vi "Page_Source_Add.vi"(4 "ctlReferences":T2, 6 "sourceInclusion":T1, 7 "items to add in":string[](array[string]), 8 "error in (no error)":errorcluster, 9 "send to main dest?":bool, 10 "Project Refnum":refnum<vi>, 11 "AB_Source_Library in":refnum<class "AB_Source_Library.lvclass">) -> (0 "error out":errorcluster, 2 "changed":bool, 3 "AB_Source_Library out":refnum<class "AB_Source_Library.lvclass">, 5 "items to add out":string[](array[string]))   [LabVIEW 2020, in "AB_Source_Library.lvclass"]
uses:
  <vilib>/AppBuilder/AB_Classes/Source/Library/AB_Source_Library.lvclass
  e:/builds/penguin/labview/branches/2020/dev/dist/vi.lib/AppBuilder/AB_Classes/Source/AB_Source.lvclass
  <resource>/Framework/Providers/Builds/AppBuilder/AB_UI_Page_Source_Files_References.ctl
  <vilib>/AppBuilder/AB_Source_Inclusion.ctl
  <vilib>/AppBuilder/AB_Classes/Source/Library/AB_Source_Library.lvclass/AB_Source_Library.ctl
  <vilib>/AppBuilder/AB_Classes/Source/AB_Source.lvclass
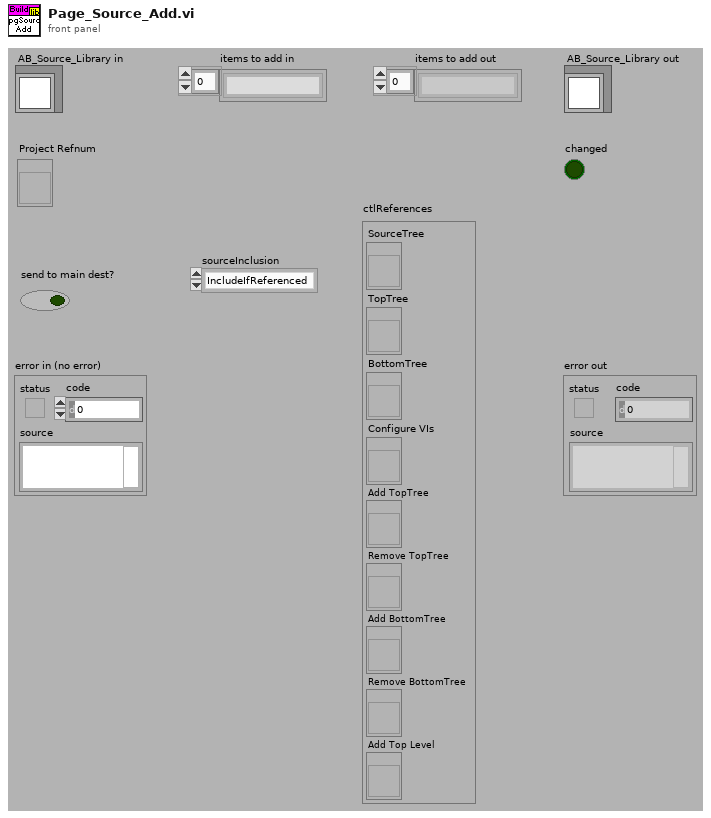
[diagram p1: front panel]
types:
  T1 = typedef "AB_Source_Inclusion.ctl" = enum16{"IncludeIfReferenced", "Include", "Exclude", "TopLevel"}
  T2 = typedef "AB_UI_Page_Source_Files_References.ctl" = cluster{"SourceTree":refnum<vi>, "TopTree":refnum<vi>, "BottomTree":refnum<vi>, "Configure VIs":refnum<vi>, "Add TopTree":refnum<vi>, "Remove TopTree":refnum<vi>, "Add BottomTree":refnum<vi>, "Remove BottomTree":refnum<vi>, "Add Top Level":refnum<vi>}
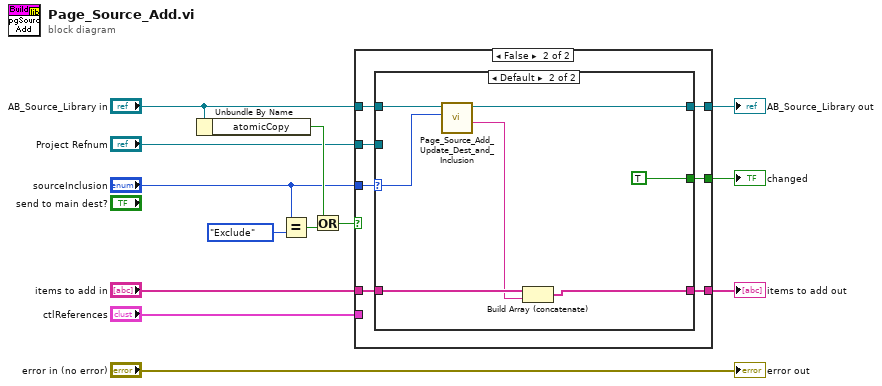
[diagram p0: block diagram]
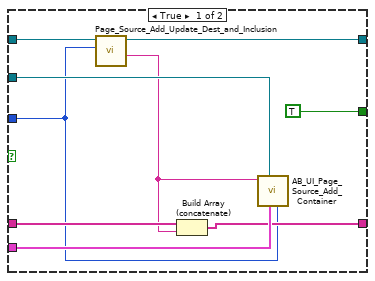
[diagram p2: hidden frame]
diagram:
  n1 = Unbundle By Name("AB_Source_Library in") -> ("atomicCopy"=w11:bool)
  n2 = Equal?(x="sourceInclusion", y=AB_Source_Inclusion."Exclude") -> (x = y?=w10:bool)
  n3 = Or(x=w11, y=w10) -> (x .or. y?=w9:bool)
  n4 = case shown="False" w9 {
    tunnel: "AB_Source_Library in" -> [w17 w29]
    tunnel: [w16 w28] -> w7
    tunnel: "ctlReferences" -> [w22 _]
    tunnel: "sourceInclusion" -> [w14 w26]
    tunnel: "Project Refnum" -> [w21 w27]
    tunnel: [TRUE w25] -> w4
    tunnel: "items to add in" -> [w19 w24]
    tunnel: [w18 w23] -> w2
    frame True {
      n5 = call <vilib>:"Page_Source_Add_Update_Dest_and_Inclusion.vi"("Inclusion"=w14, "AB_Source_VI in"=w17) -> ("itemID"=w15:string, "AB_Source_VI out"=w16:refnum<class "AB_Source_Library.lvclass">)  [unwired: 7 in, 1 out]
      n6 = Build Array (concatenate)(w19, w15) -> (w18:string[])
      n7 = call <resource>:"AB_UI_Page_Source_Add_Container.vi"("sourceInclusion"=w14, "ctlReferences"=w22, "Project Refnum"=w21, "itemID"=w15) -> ()  [unwired: 7 in, 1 out]
    }
    frame False {
      n8 = case shown="Default" w26 {
        selector: w26 -> [_ w32]
        tunnel: w29 -> [w31 w35]
        tunnel: [w31 w34] -> w28
        tunnel: w27 -> [_ _]
        tunnel: [_ TRUE] -> w25
        tunnel: w24 -> [w30 w37]
        tunnel: [w30 w36] -> w23
        frame "TopLevel" {
        }
        frame Default {
          n9 = call <vilib>:"Page_Source_Add_Update_Dest_and_Inclusion.vi"("Inclusion"=w32, "AB_Source_VI in"=w35) -> ("itemID"=w33:string, "AB_Source_VI out"=w34:refnum<class "AB_Source_Library.lvclass">)  [unwired: 7 in, 1 out]
          n10 = Build Array (concatenate)(w37, w33) -> (w36:string[])
        }
      }
    }
  }
  "changed" <- w4
  "AB_Source_Library out" <- w7
  "items to add out" <- w2
  "error out" <- "error in (no error)"
